vi "Set Instrument Database.vi"(8 "error in (no error)":errorcluster caption="entrée d'erreur (pas d'erreur)", 10 "Library Instruments.lvlib:Class Instrument (Default).lvclass":refnum<class "Class Instrument (Default).lvclass">, 11 "Creation_SN Database (Default) en entrée":refnum<class "Creation_SN Database (Default).lvclass">) -> (0 "error out":errorcluster caption="sortie d'erreur", 3 "Creation_SN Database (Default) en sortie":refnum<class "Creation_SN Database (Default).lvclass">)   [LabVIEW 2020, in "Library Instrument & Equipement.lvlib" / "Library Creation_SN.lvlib" / "Creation_SN Database (Default).lvclass"]
uses:
  Creation_SN Database (Default).lvclass
  Instrument/Instrument (Default)/Class Instrument (Default).lvclass
  Creation_SN Database (Default).lvclass/Creation_SN Database (Default).ctl
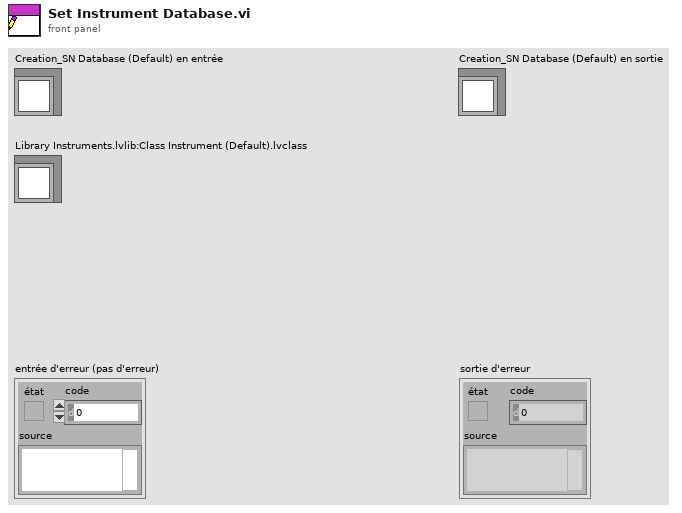
[diagram p1: front panel]
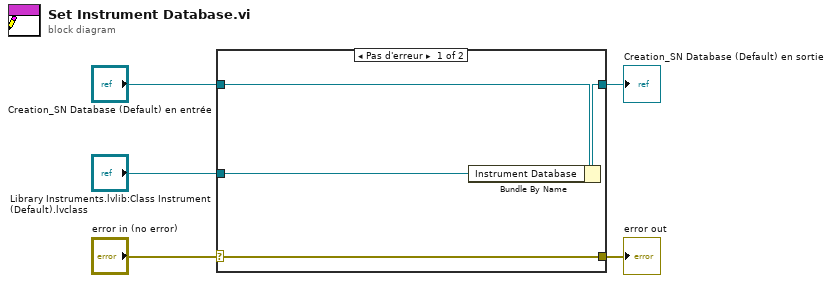
[diagram p0: block diagram]
diagram:
  n1 = case shown="Pas d'erreur" "error in (no error)" {
    selector: "error in (no error)" -> [w9 w10]
    tunnel: [w9 w10] -> w4
    tunnel: [w7 w11] -> w2
    tunnel: "Creation_SN Database (Default) en entrée" -> [w8 w11]
    tunnel: "Library Instruments.lvlib:Class Instrument (Default).lvclass" -> [w6 _]
    frame No Error {
      n2 = Bundle By Name(cluster=w8, "Instrument Database"=w6) -> (w7:refnum<class "Creation_SN Database (Default).lvclass">)
    }
    frame Error {
    }
  }
  "error out" <- w4
  "Creation_SN Database (Default) en sortie" <- w2
